vi "NI VeriStand - Commit System Explorer Update Buffer.vi"(8 "error in (no error)":errorcluster) -> (0 "error out":errorcluster)   [LabVIEW 2020, in "Custom Device API.lvlib"]
doc: "Commits updates to the <B>System Explorer</B> window. Using this VI together with the Enable System Explorer Update Buffer VI can speed up item creation if you are creating or updating multiple custom device items at one time."
uses:
  <vilib>/NI VeriStand/Custom Device API/Custom Device API.lvlib
  584c7e3e-3fc6-4c42-9e11-3b2deab15229.vi
  <vilib>/NI VeriStand/Custom Device API/Custom Device Offline Path.vi
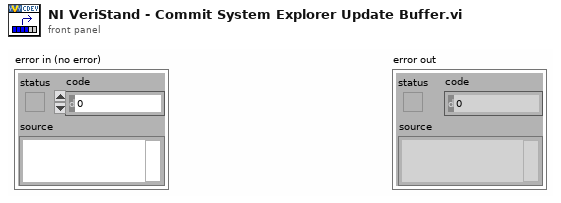
[diagram p1: front panel]
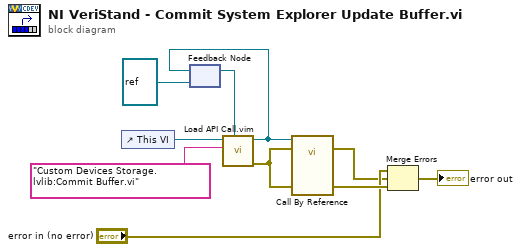
[diagram p0: block diagram]
diagram:
  n1 = control-ref of="This VI"() -> (w7:refnum<vi>)
  n2 = feedback #1(refnum<vi> refnum ("type specifier VI Refnum (for type only)")) -> (w8:refnum<vi>)
  n3 = call "Load API Call.vim"("VI reference in"=w8, "VI qualified name"="Custom Devices Storage.lvlib:Commit Buffer.vi", "Caller VI ref"=w7) -> ("error out"=w5:errorcluster, "VI reference"=w4:refnum<vi>)  [unwired: 7 in]
  n4 = feedback-in #1(w4) -> ()
  n5 = call-by-ref "?"(reference=w4, error in=w5, 8:"error in (no error)"=w5) -> (error out=w1:errorcluster, 0:"error out"=w10:errorcluster)  [unwired: 10 in, 1 out]
  n6 = Merge Errors("error in (no error)", w1, w10) -> (→"error out":errorcluster)
